vi "Test LRS FPGA.vi"() -> ()   [LabVIEW 2014]
uses:
  <vilib>/rvi/Emulation/niFpgaGetClockAttributes.vi
  <vilib>/rvi/Emulation/niFpgaSctlEmulationGetInTimedLoop.vi
  <vilib>/rvi/Emulation/niFpgaEmulationReportErrorSimple.vi
  <vilib>/rvi/Emulation/niFpgaProcessEmulError.vi
  <vilib>/rvi/interface/RandomDataEmulation/niFpgaRandomDataHandleErrors.vi
  <vilib>/rvi/Emulation/niFpgaCriticalErrorInLSC.vi
  <vilib>/rvi/DataTransferAndStorage/Container/XNode/niFpgaContainer.xnode
  <vilib>/rvi/interface/RandomDataEmulation/nirviRandomDataFpgaReadWriteTemplate.vi
panel:
  out "L":fxp<+,64,57>[](array[numeric]) format="%.25g"
  in  "Num2Proc":i32
  in  "Start Calc":bool=TRUE
  in  "Stop":bool
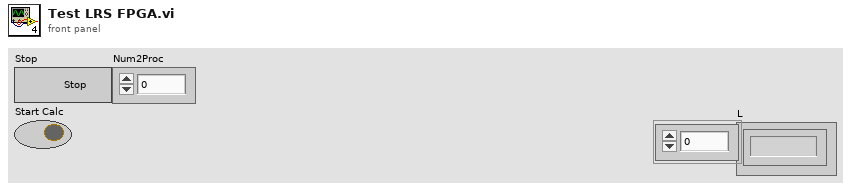
[diagram p1: front panel]
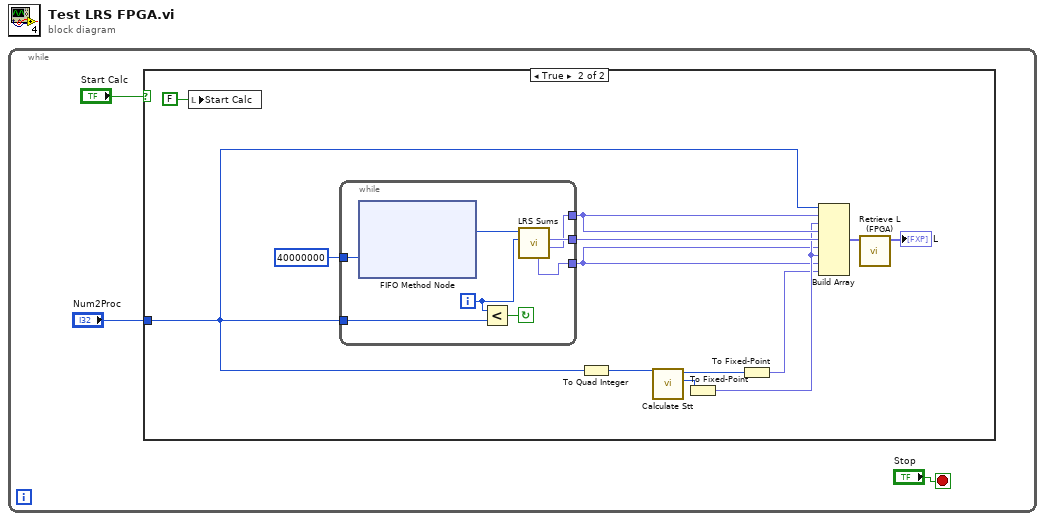
[diagram p0: block diagram]
diagram:
  n1 = while {
    stop <- "Stop" stop-if-true
    n2 = case shown="True" "Start Calc" {
      tunnel: "Num2Proc" -> [_ w10]
      frame False {
      }
      frame True {
        n3 = local write "Start Calc"(FALSE ("Start Calc")) -> ()
        n4 = while {
          tunnel: w10 -> [w24]
          tunnel: [w20] -> w8
          tunnel: [w19] -> w9
          tunnel: [w18] -> w6
          tunnel: 40000000 ("Timeout") -> [w17]
          i -> [w21]
          stop <- w23 continue-if-true
          n5 = xnode ("FIFO Method Node")("Timeout"=w17) -> ("Element"=w22:i16)  [unwired: 1 in, 2 out]
          n6 = Less?(x=w21, y=w24) -> (x < y?=w23:bool)
          n7 = call "LRS Sums.vi"("i"=w21, "DataIn"=w22) -> ("SI"=w19:fxp<+,40,40>, "SII"=w20:fxp<+,64,64>, "StI"=w18:fxp<+,54,54>)  [unwired: 4 in, 3 out]
        }
        n8 = To Quad Integer(1:w10) -> (0:w14:i64)
        n9 = call "Calculate Stt.vi"("N"=w14) -> ("St"=w11:i64, "Stt"=w12:i64)  [unwired: 9 in]
        n10 = To Fixed-Point(number=w11) -> (fixed-point=w7:fxp<+/-,64,64>)  [unwired: 1 in]
        n11 = To Fixed-Point(number=w12) -> (fixed-point=w5:fxp<+/-,64,64>)  [unwired: 1 in]
        n12 = Build Array(w10, w9, w7, w9, w8, w6, w7, w6, w5) -> (w4:fxp<+/-,64,65>[])
        n13 = call "Retrieve L (FPGA).vi"("Matrix In"=w4) -> ("L"=→"L":fxp<+,64,57>[])  [unwired: 9 in]
      }
    }
  }
